vi "Bus Controller Suite.vi"   [LabVIEW 2020, in "Unit Tests.lvlib"]
uses:
  Unit Tests.lvlib
  Tests/Bus Controller/Bus Controller.lvclass
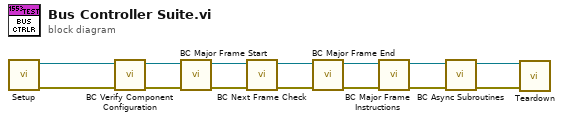
[diagram p0: block diagram]
diagram:
  n1 = call "Setup.vi"() -> ("error out"=w14:errorcluster, "Bus Controller out"=w13:refnum<class "Bus Controller.lvclass">)  [unwired: 10 in]
  n2 = call "BC Verify Component Configuration.vi"("error in (no error)"=w14, "Bus Controller in"=w13) -> ("error out"=w4:errorcluster, "Bus Controller out"=w3:refnum<class "Bus Controller.lvclass">)  [unwired: 8 in]
  n3 = call "BC Major Frame Start.vi"("error in (no error)"=w4, "Bus Controller in"=w3) -> ("error out"=w6:errorcluster, "Bus Controller out"=w5:refnum<class "Bus Controller.lvclass">)  [unwired: 8 in]
  n4 = call "BC Next Frame Check.vi"("error in (no error)"=w6, "Bus Controller in"=w5) -> ("error out"=w8:errorcluster, "Bus Controller out"=w7:refnum<class "Bus Controller.lvclass">)  [unwired: 8 in]
  n5 = call "BC Major Frame End.vi"("error in (no error)"=w8, "Bus Controller in"=w7) -> ("error out"=w10:errorcluster, "Bus Controller out"=w9:refnum<class "Bus Controller.lvclass">)  [unwired: 8 in]
  n6 = call "BC Major Frame Instructions.vi"("error in (no error)"=w10, "Bus Controller in"=w9) -> ("error out"=w2:errorcluster, "Bus Controller out"=w1:refnum<class "Bus Controller.lvclass">)  [unwired: 8 in]
  n7 = call "BC Async Subroutines.vi"("error in (no error)"=w2, "Bus Controller in"=w1) -> ("error out"=w11:errorcluster, "Bus Controller out"=w12:refnum<class "Bus Controller.lvclass">)  [unwired: 8 in]
  n8 = call "Teardown.vi"("error in (no error)"=w11, "Bus Controller in"=w12) -> ()  [unwired: 9 in, 1 out]
